vi "send PIE (with CW).vi"() -> ()   [LabVIEW 2017]
uses:
  <instrlib>/niUSRP/niUSRP Write Tx Data (CDB).vi
  <vilib>/measure/NI_MABase.lvlib
panel:
  in  "停止":bool
  out "波形图":dbl[](graph)
  out "0":waveform(dbl)(graph)
  out "error out":errorcluster
  in  "end of data?":bool
  in  "timeout":dbl=10.0
  out "coerced IQ rate":dbl=100000.0 format="%#_6p"
  out "coerced gain":dbl format="%#_6f"
  out "coerced carrier frequency":dbl=100000.0 format="%#_6p"
  in  "active antenna":string="TX1"
  in  "gain":dbl=30.0 format="%#_6f"
  in  "carrier frequency":dbl=915000000.0 format="%#_6p"
  in  "IQ rate":dbl=1000000.0 format="%#_6p"
  in  "Enabled Channels":string="0"
  in  "device names":refnum<k15>="192.168.10.10"
  in  "signal type 2":T1(ring)=enum."Square Wave" caption="信号类型"
  in  "amplitude 2":dbl=0.707 caption="幅值" format="%#.6g"
  in  "square wave duty cycle (%) 2":dbl=95.238 caption="方波占空比(%)" format="%0.2f"
  in  "单个周期持续时间(s) 2":dbl=0.000105 format="%#_13g"
  out "字符串":string="信号1设置"
  in  "signal type 3":T1(ring)=enum."Square Wave" caption="信号类型"
  in  "amplitude 3":dbl=0.707 caption="幅值" format="%#.6g"
  in  "square wave duty cycle (%) 3":dbl=97.5609 caption="方波占空比(%)" format="%0.2f"
  out "1":waveform(dbl)(graph)
  in  "单个周期持续时间(s)":dbl=0.000205 format="%#_13g"
  out "?":string="信号0设置"
  out "大小":i32
  in  "输入序列":u32[](array[numeric]) format="%b"
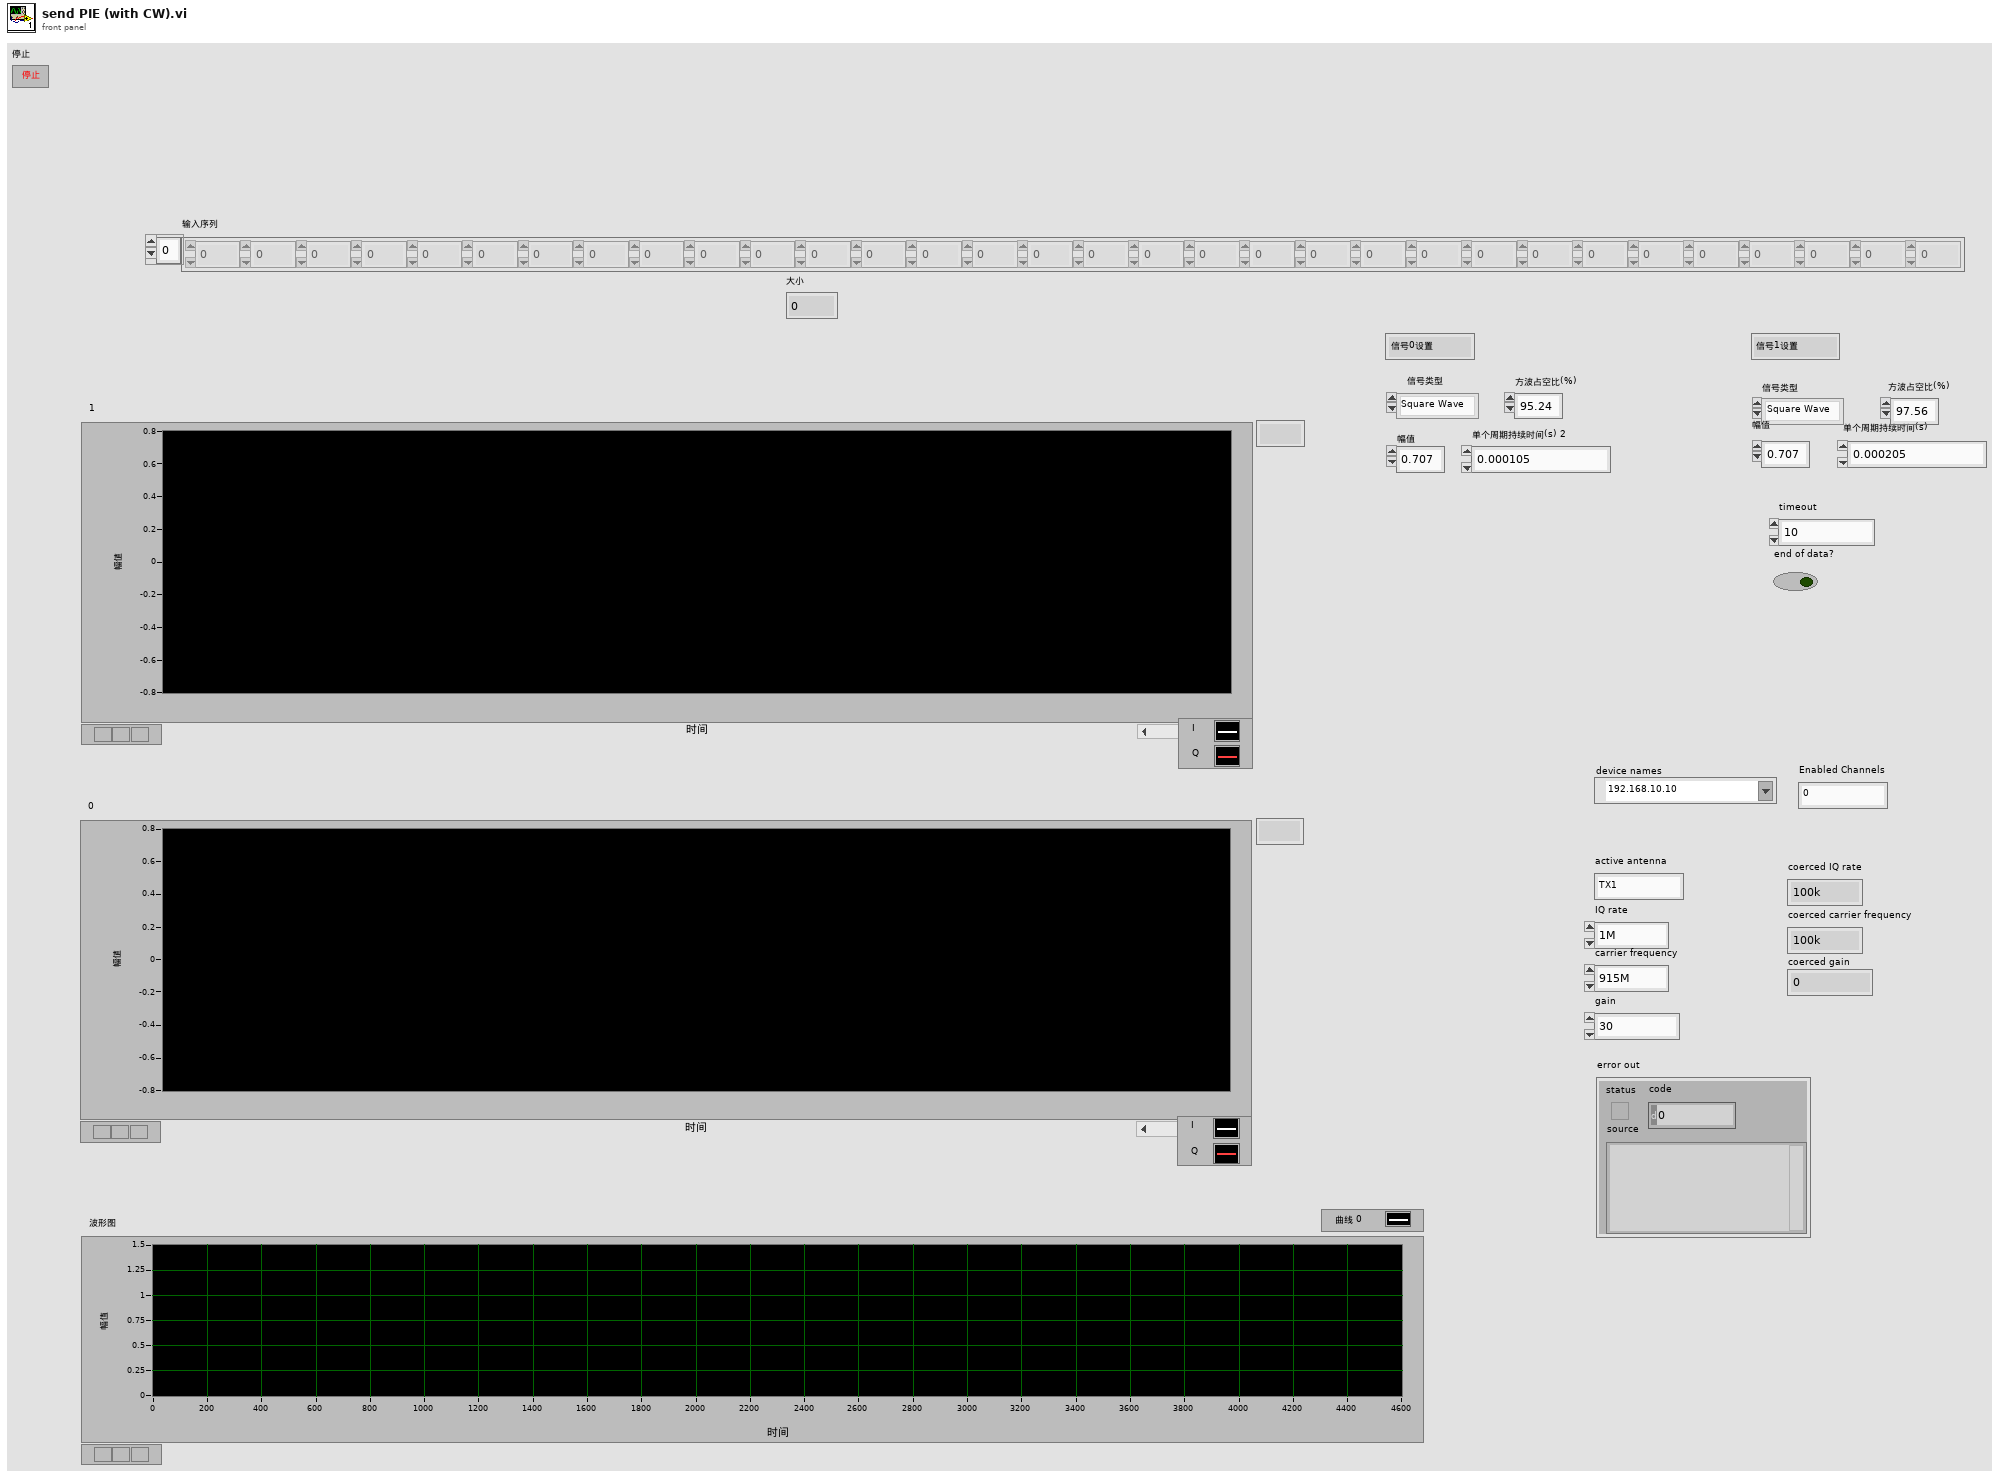
[diagram p1: front panel]
types:
  T1 = enum16{"Sine Wave", "Triangle Wave", "Square Wave", "Sawtooth Wave"}
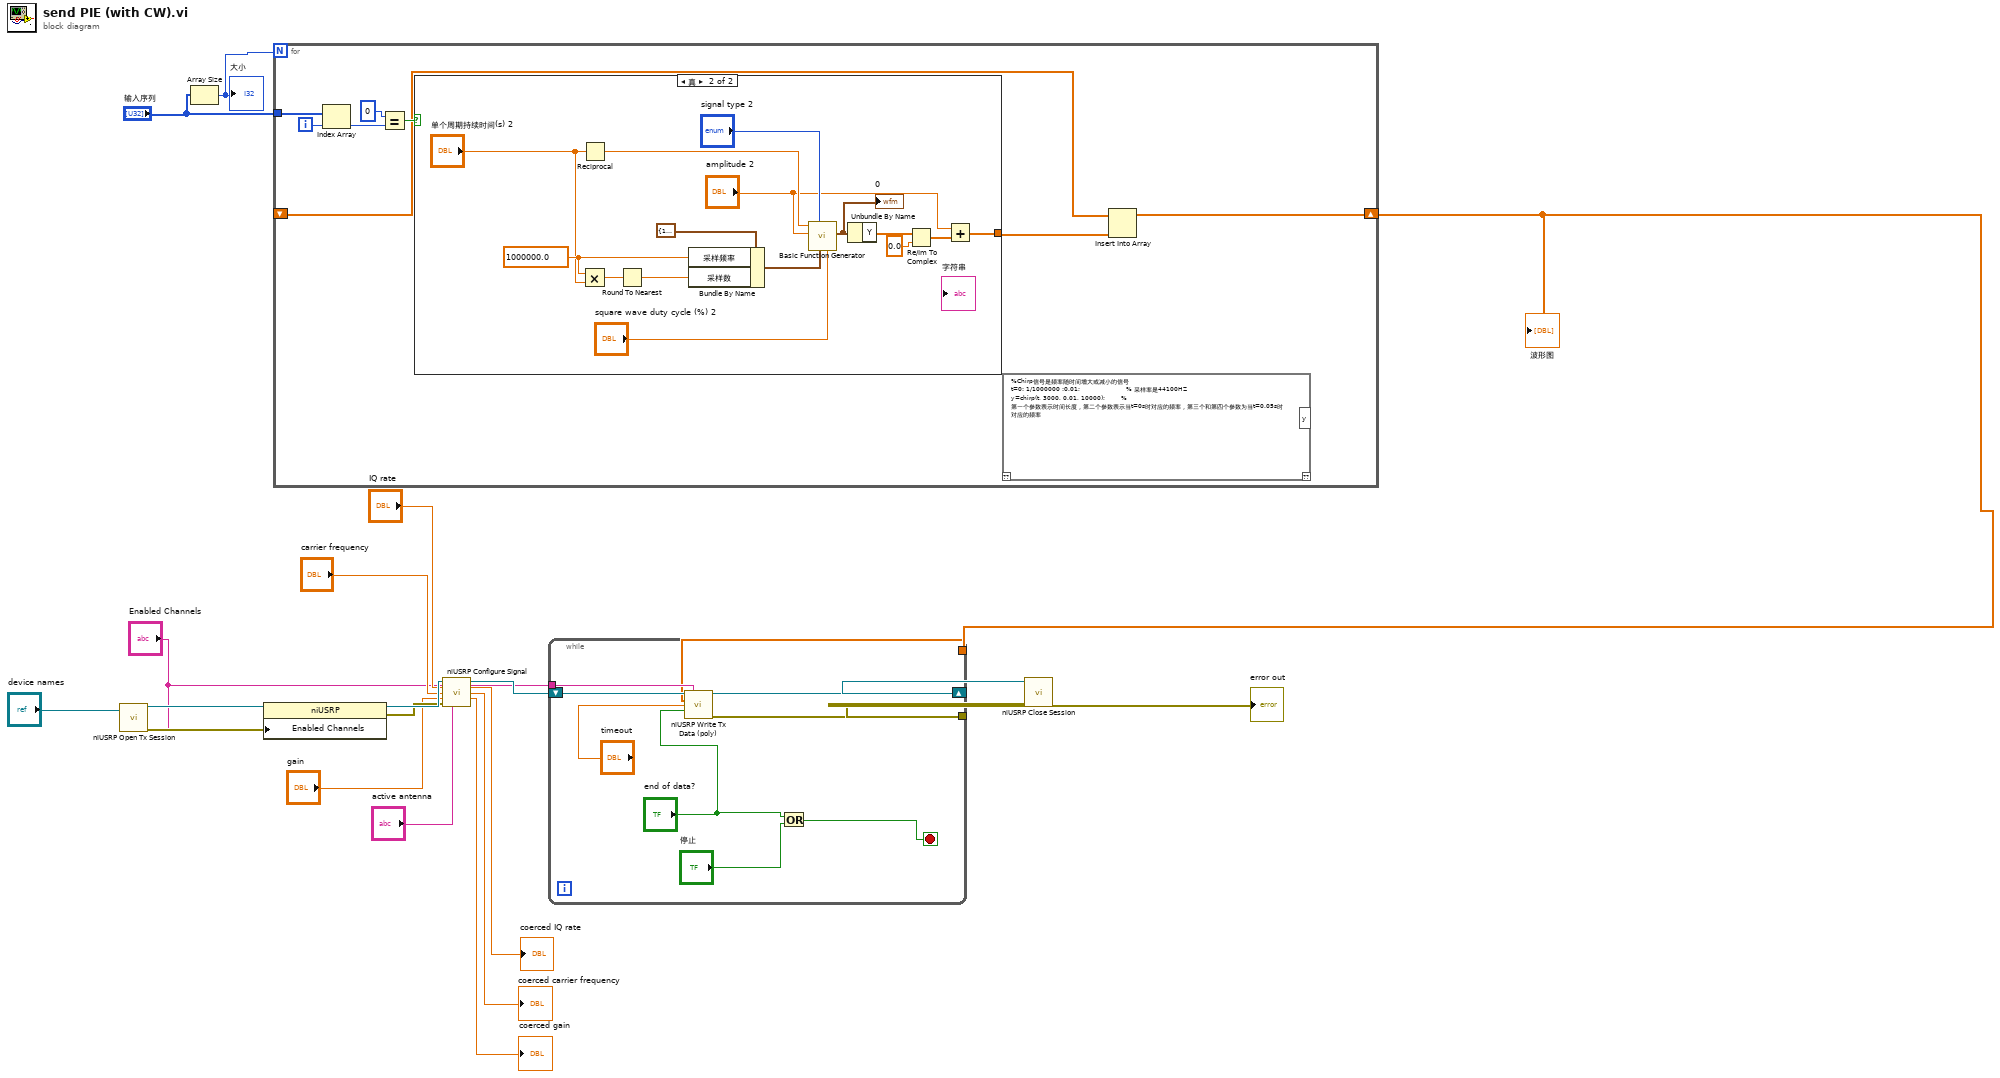
[diagram p0: block diagram]
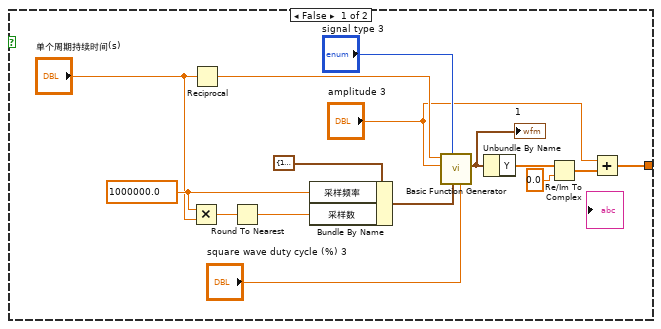
[diagram p2: hidden frame]
diagram:
  n1 = call <instrlib>:"niUSRP Open Tx Session.vi"("device names"="device names") -> ("session handle out"=w17:refnum<k15>, "error out"=w16:errorcluster)  [unwired: 13 in]
  n2 = Array Size(array="输入序列") -> (size(s)=w20:i32)
  "大小" <- w20
  n3 = property class="niUSRP"(reference=w17, error in=w16, "Enabled Channels"="Enabled Channels") -> (reference out=w15:refnum<k15>, error out=w14:errorcluster)
  n4 = for {
    N: w20 -> [_]
    tunnel: "输入序列" -> [w25]
    shift-right: [w23] -> w1
    shift-left: _ -> [w22]
    i -> [w28]
    n5 = Index Array(array=w25, index=w28) -> (element=w24:u32)
    n6 = Equal?(x=u32 0, y=w24) -> (x = y?=w26:bool)
    n7 = case shown="真" w26 {
      tunnel: [w32 w47] -> w21
      frame False {
        w41 = 1000000.0 ("采样频率")
        n8 = Multiply(x=w41, y="单个周期持续时间(s)") -> (x*y=w42:dbl)
        n9 = Reciprocal(x="单个周期持续时间(s)") -> (1/x=w35:dbl)
        n10 = Round To Nearest(number=w42) -> (nearest integer value=w39:dbl)
        n11 = Bundle By Name ("按名称捆绑")(cluster=cluster{"采样频率":dbl, "采样数":i32} {"采样频率"=1000000.0, "采样数"=1000}, "采样频率"=w41, "采样数"=w39) -> (w37:cluster{"采样频率":dbl, "采样数":i32})
        n12 = call <vilib>:"Basic Function Generator.vi"("square wave duty cycle (%)"="square wave duty cycle (%) 3", "sampling info"=w37, "signal type"="signal type 3", "amplitude"="amplitude 3", "frequency"=w35) -> ("signal out"=w29:waveform(dbl))  [unwired: 4 in, 2 out]
        "1" <- w29
        n13 = Unbundle By Name(w29) -> ("Y"=w34:dbl[])
        n14 = Re/Im To Complex(1:0.0, 2:w34) -> (0:w31:cdb[])
        n15 = Add(x="amplitude 3", y=w31) -> (x+y=w32:cdb[])
      }
      frame True {
        w53 = 1000000.0 ("采样频率")
        n16 = Multiply(x=w53, y="单个周期持续时间(s) 2") -> (x*y=w52:dbl)
        n17 = Reciprocal(x="单个周期持续时间(s) 2") -> (1/x=w54:dbl)
        n18 = Round To Nearest(number=w52) -> (nearest integer value=w51:dbl)
        n19 = Bundle By Name ("按名称捆绑")(cluster=cluster{"采样频率":dbl, "采样数":i32} {"采样频率"=1000000.0, "采样数"=1000}, "采样频率"=w53, "采样数"=w51) -> (w57:cluster{"采样频率":dbl, "采样数":i32})
        n20 = call <vilib>:"Basic Function Generator.vi"("square wave duty cycle (%)"="square wave duty cycle (%) 2", "sampling info"=w57, "signal type"="signal type 2", "amplitude"="amplitude 2", "frequency"=w54) -> ("signal out"=w44:waveform(dbl))  [unwired: 4 in, 2 out]
        "0" <- w44
        n21 = Unbundle By Name(w44) -> ("Y"=w46:dbl[])
        n22 = Re/Im To Complex(1:0.0, 2:w46) -> (0:w49:cdb[])
        n23 = Add(x="amplitude 2", y=w49) -> (x+y=w47:cdb[])
      }
    }
    n24 = script code="%Chirp信号是频率随时间增大或减小的信号\nt=0: 1/1000000 :0.01;                       % 采样率是44100HZ\ny=chirp(t, 3000, 0.01, 10000);        % 第一个参数表示时间长度，第二个参数表示当t=0s时对应的频率，第三个和第四个参数为当t=0.05s时对应的频率"() -> ()  [unwired: 1 in, 2 out]
    n25 = Insert Into Array(array=w22, new element=w21) -> (w23:cdb[])  [unwired: 1 in]
  }
  "波形图" <- w1
  n26 = call <instrlib>:"niUSRP Configure Signal.vi"("session handle"=w15, "channel list"="Enabled Channels", "IQ rate"="IQ rate", "carrier frequency"="carrier frequency", "gain"="gain", "error in (no error)"=w14, "active antenna"="active antenna") -> ("session handle out"=w6:refnum<k15>, "coerced IQ rate"=→"coerced IQ rate":dbl, "coerced carrier frequency"=→"coerced carrier frequency":dbl, "coerced gain"=→"coerced gain":dbl)  [unwired: 4 in, 1 out]
  n27 = while {
    tunnel: "Enabled Channels" -> [w66]
    tunnel: [w63] -> w2
    tunnel: w1 -> [w62]
    shift-right: [w64] -> w3
    shift-left: w6 -> [w67]
    stop <- w59 stop-if-true
    n28 = call-poly <instrlib>:"niUSRP Write Tx Data (poly).vi"("session handle"=w67, "channel list"=w66, "data"=w62, "timeout"="timeout", "end of data?"="end of data?") -> ("session handle out"=w64:refnum<k15>, "error out"=w63:errorcluster)  [unwired: 9 in]
    n29 = Or(x="end of data?", y="停止") -> (x .or. y?=w59:bool)
  }
  n30 = call <instrlib>:"niUSRP Close Session.vi"("session handle"=w3, "error in (no error)"=w2) -> ("error out"=→"error out":errorcluster)  [unwired: 13 in]
